vi "disable fp elements during scanning.vi"(11 "T for grey out":bool) -> ()   [LabVIEW 2017]
doc: "SciScan 1.2 160622"
uses:
  GFG/GFGfpRefGet.vi
  GFG/GFG library.lvlib
panel:
  out "error out 3":errorcluster
  out "error out 2":errorcluster
  out "error out":errorcluster
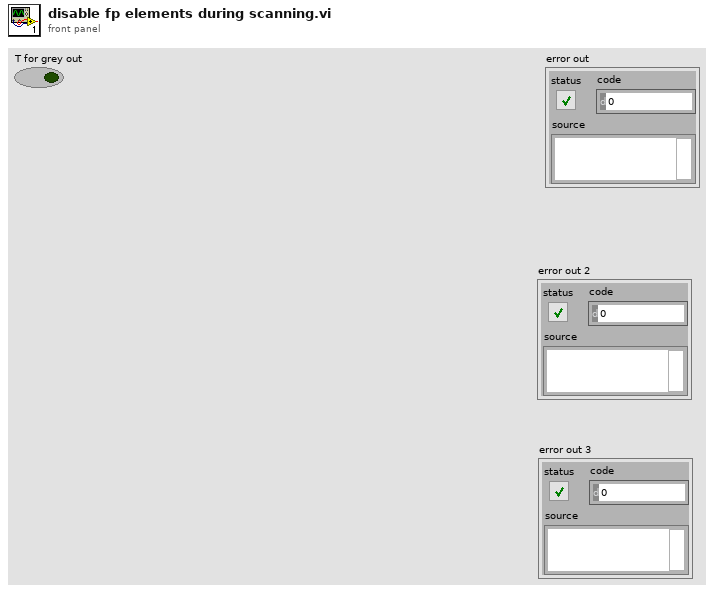
[diagram p1: front panel]
types:
  T1 = enum8{"Enabled", "Disabled", "Disabled and Grayed Out"}
  T2 = cluster{"WaveformChartRef":refnum<vi>, "DigitalRef":refnum<vi>, "ArrayRef":refnum<vi>, "TabControlRef":refnum<vi>, "EnumRef":refnum<vi>, "RingRef":refnum<vi>, "BooleanRef":refnum<vi>, "KnobRef":refnum<vi>, "SlideRef":refnum<vi>, "PathRef":refnum<vi>, "StringRef":refnum<vi>, "ComboBox":refnum<vi>, "WaveformGraphRef":refnum<vi>}
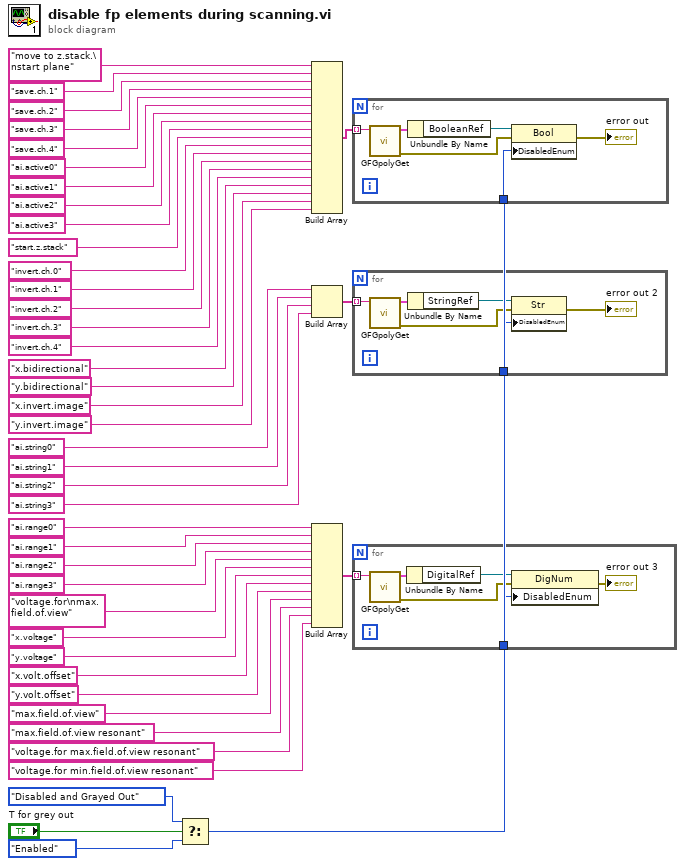
[diagram p0: block diagram]
diagram:
  n1 = Select(t=T1."Disabled and Grayed Out" ("Disabled"), s="T for grey out", f=T1."Enabled" ("Disabled")) -> (s? t:f=w19:T1)
  n2 = Build Array("move to z.stack.\nstart plane" ("element"), "save.ch.1" ("Variable Name in"), "save.ch.2" ("Variable Name in"), "save.ch.3" ("Variable Name in"), "save.ch.4" ("Variable Name in"), "ai.active0" ("Variable Name in"), "ai.active1" ("Variable Name in"), "ai.active2" ("Variable Name in"), "ai.active3" ("Variable Name in"), "start.z.stack" ("Variable Name in"), "invert.ch.0" ("Variable Name in"), "invert.ch.1" ("Variable Name in"), "invert.ch.2" ("Variable Name in"), "invert.ch.3" ("Variable Name in"), "invert.ch.4" ("Variable Name in"), "x.bidirectional" ("Variable Name in"), "y.bidirectional" ("Variable Name in"), "x.invert.image" ("Variable Name in"), "y.invert.image" ("Variable Name in")) -> (w31:string[])
  n3 = Build Array("ai.string0" ("Variable Name in"), "ai.string1" ("Variable Name in"), "ai.string2" ("Variable Name in"), "ai.string3" ("Variable Name in")) -> (w20:string[])
  n4 = Build Array("ai.range0" ("Variable Name in"), "ai.range1" ("Variable Name in"), "ai.range2" ("Variable Name in"), "ai.range3" ("Variable Name in"), "voltage.for\nmax.field.of.view" ("Variable Name in"), "x.voltage" ("Variable Name in"), "y.voltage" ("Variable Name in"), "x.volt.offset" ("Variable Name in"), "y.volt.offset" ("Variable Name in"), "max.field.of.view" ("Variable Name in"), "max.field.of.view resonant" ("Variable Name in"), "voltage.for max.field.of.view resonant" ("Variable Name in"), "voltage.for min.field.of.view resonant" ("Variable Name in")) -> (w14:string[])
  n5 = for {
    tunnel: w19 -> [w47]
    tunnel: w31 -> [w46] mode=indexing
    n6 = call-poly "GFGpolyGet.vi"("Variable Name in"=w46) -> ("error out"=w45:errorcluster, "output cluster"=w49:T2)  [unwired: 9 in]
    n7 = Unbundle By Name(w49) -> ("BooleanRef"=w48:refnum<vi>)
    n8 = property class="Bool"(reference=w48, error in=w45, "DisabledEnum"=w47) -> (error out=→"error out":errorcluster)  [unwired: 1 out]
  }
  n9 = for {
    tunnel: w19 -> [w53]
    tunnel: w20 -> [w52] mode=indexing
    n10 = call-poly "GFGpolyGet.vi"("Variable Name in"=w52) -> ("error out"=w51:errorcluster, "output cluster"=w55:T2)  [unwired: 9 in]
    n11 = Unbundle By Name(w55) -> ("StringRef"=w54:refnum<vi>)
    n12 = property class="Str"(reference=w54, error in=w51, "DisabledEnum"=w53) -> (error out=→"error out 2":errorcluster)  [unwired: 1 out]
  }
  n13 = for {
    tunnel: w19 -> [w59]
    tunnel: w14 -> [w58] mode=indexing
    n14 = call-poly "GFGpolyGet.vi"("Variable Name in"=w58) -> ("error out"=w57:errorcluster, "output cluster"=w61:T2)  [unwired: 9 in]
    n15 = Unbundle By Name(w61) -> ("DigitalRef"=w60:refnum<vi>)
    n16 = property class="DigNum"(reference=w60, error in=w57, "DisabledEnum"=w59) -> (error out=→"error out 3":errorcluster)  [unwired: 1 out]
  }
